vi "Measure RPM.vi"(5 "Active":bool, 7 "number of samples per channel":i32=1000, 8 "error in":errorcluster, 10 "timeout":dbl=0.05 format="%#_13g", 11 "Knob in":refnum<vi>) -> (0 "error out":errorcluster, 2 "Raw":dbl[](array[numeric]) format="%0.2f", 3 "Mean RPM":dbl format="%0.2f")   [LabVIEW 2017]
uses:
  <vilib>/DAQmx/read.llb/DAQmx Read (Counter 1D DBL 1Chan NSamp).vi
  <vilib>/Analysis/baseanly.llb/Mean (DBL).vi
  <vilib>/DAQmx/miscellaneous.llb/DAQmx Fill In Error Info.vi
  <vilib>/Analysis/NI_AALBase.lvlib
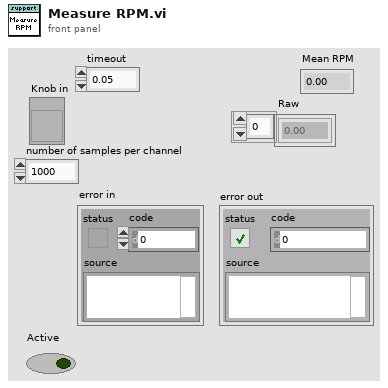
[diagram p1: front panel]
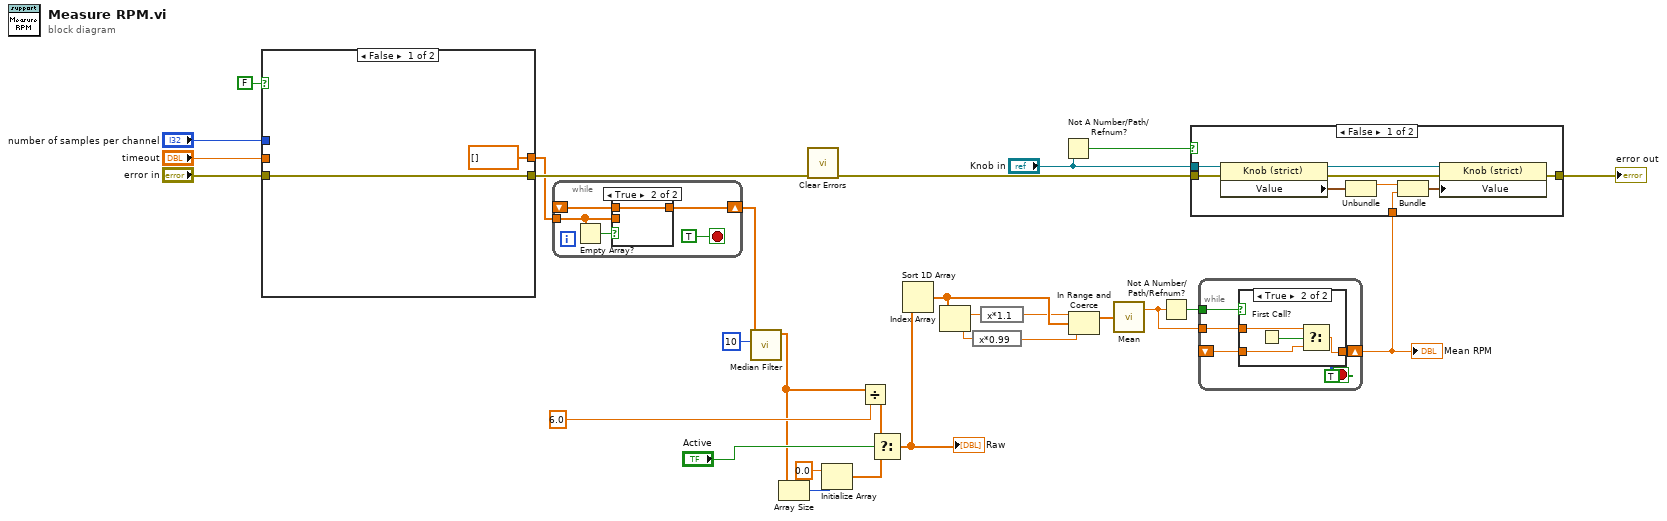
[diagram p0: block diagram]
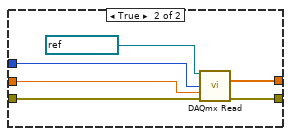
[diagram p2: hidden frame]
diagram:
  n1 = case shown="False" FALSE {
    tunnel: [w30 w36] -> w28
    tunnel: "error in" -> [w30 w34]
    tunnel: "number of samples per channel" -> [_ w33]
    tunnel: "timeout" -> [_ w32]
    tunnel: [dbl[] [] ("data") w31] -> w12
    frame False {
    }
    frame True {
      n2 = call-poly <vilib>:"DAQmx Read.vi"("task/channels in"=refnum<k21> "PrecorDI", "number of samples per channel"=w33, "timeout"=w32, "error in"=w34) -> ("data"=w31:dbl[], "error out"=w36:errorcluster)  [unwired: 9 in, 1 out]
    }
  }
  n3 = while {
    tunnel: w12 -> [w39]
    shift-right: [w40] -> w4
    shift-left: _ -> [w38]
    stop <- TRUE stop-if-true
    n4 = Empty Array?(array=w39) -> (empty?=w41:bool)
    n5 = case shown="True" w41 {
      tunnel: [w42 w43] -> w40
      tunnel: w39 -> [w42 _]
      tunnel: w38 -> [_ w43]
      frame False {
      }
      frame True {
      }
    }
  }
  n6 = call <vilib>:"Median Filter.vi"("left rank"=10, "X"=w4) -> ("Filtered X"=w3:dbl[])  [unwired: 8 in, 1 out]
  n7 = Array Size(array=w3) -> (size(s)=w11:i32)
  n8 = call <vilib>:"Clear Errors.vi"("error in (no error)"=w28) -> ("error out"=w16:errorcluster)  [unwired: 5 in, 1 out]
  n9 = Initialize Array(0.0 ("element"), w11) -> (w8:dbl[])
  n10 = Divide(x=w3, y=6.0 ("frequency")) -> (x/y=w7:dbl[])
  n11 = Select(t=w7, s="Active", f=w8) -> (s? t:f=w6:dbl[])
  "Raw" <- w6
  n12 = Sort 1D Array(array=w6) -> (sorted array=w22:dbl[])
  n13 = Index Array(array=w22) -> (element=w21:dbl)  [unwired: 1 in]
  n14 = expression code="x*0.99"(w21) -> (w19:dbl)
  n15 = expression code="x*1.1"(w21) -> (w20:dbl)
  n16 = Not A Number/Path/Refnum?(number/path/refnum="Knob in") -> (NaN/Path/Refnum?=w23:bool)
  n17 = In Range and Coerce(upper limit=w20, x=w22, lower limit=w19) -> (coerced(x)=w18:dbl[])  [unwired: 1 out]
  n18 = call-poly <vilib>:"Mean.vi"("X"=w18) -> ("mean"=w14:dbl)  [unwired: 1 out]
  n19 = Not A Number/Path/Refnum?(number/path/refnum=w14) -> (NaN/Path/Refnum?=w15:bool)
  n20 = while {
    shift-right: [w47] -> w5
    shift-left: _ -> [w45]
    tunnel: w15 -> [w48]
    tunnel: w14 -> [w46]
    stop <- TRUE stop-if-true
    n21 = case shown="True" w48 {
      tunnel: [w49 w50] -> w47
      tunnel: w46 -> [w49 w52]
      tunnel: w45 -> [_ w51]
      frame False {
      }
      frame True {
        n22 = First Call?() -> (First Call?: T/F=w53:bool)
        n23 = Select(t=w52, s=w53, f=w51) -> (s? t:f=w50:dbl)
      }
    }
  }
  "Mean RPM" <- w5
  n24 = case shown="False" w23 {
    tunnel: w16 -> [w61 w63]
    tunnel: w5 -> [w56 _]
    tunnel: [w55 w63] -> w26
    tunnel: "Knob in" -> [w54 _]
    frame False {
      n25 = property class="Knob (strict)"(reference=w54, error in=w61) -> (reference out=w58:refnum<vi>, error out=w57:errorcluster, "Value"=w60:cluster{dbl, dbl})
      n26 = Unbundle(w60) -> (w62:dbl)  [unwired: 1 out]
      n27 = Bundle(w62, "mean"=w56) -> (w59:cluster{dbl, "mean":dbl})  [unwired: 1 in]
      n28 = property class="Knob (strict)"(reference=w58, error in=w57, "Value"=w59) -> (error out=w55:errorcluster)  [unwired: 1 out]
    }
    frame True {
    }
  }
  "error out" <- w26
